vi "read_config_file.vi"(8 "error in (no error)":errorcluster, 10 "force load?":bool, 11 "StageMG100204SutterMP285 in":refnum<class "StageMG100204SutterMP285.lvclass">=refnum) -> (0 "error out":errorcluster, 3 "StageMG100204SutterMP285 out":refnum<class "StageMG100204SutterMP285.lvclass">)   [LabVIEW 2010, in "StageMG100204SutterMP285.lvclass"]
doc: "The dynamic dispatch version of this VI loads the config file from the config_files folder of the actual plug-in class. The name of the config file to be loaded is property of the plug-in object. If not explicitely set, a file config_files/config.xml is loaded by default."
uses:
  StageMG100204SutterMP285.lvclass
  configuration_data_cluster.ctl
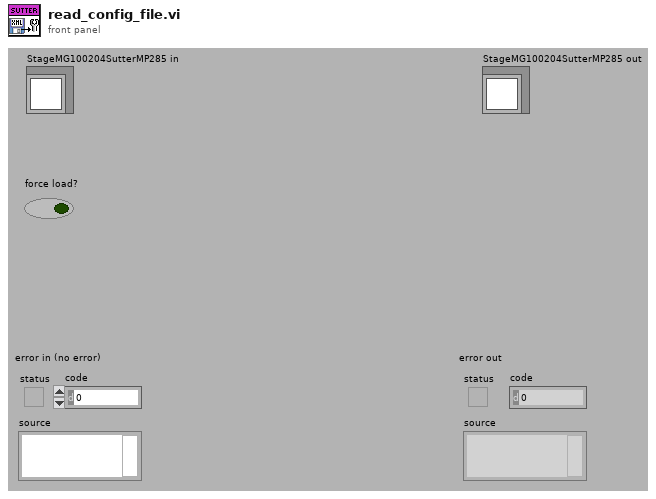
[diagram p1: front panel]
types:
  T1 = typedef "StageMG100204SutterMP285.lvclass/configuration_data_cluster.ctl" = cluster{"serial port":dbl, "HiRes Speed":dbl, "LoRes Speed":dbl}
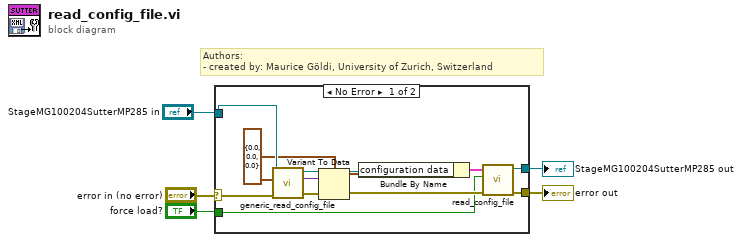
[diagram p0: block diagram]
diagram:
  # "Authors: \n- created by: Maurice Göldi, University of Zurich, Switzerland"
  n1 = case shown="No Error" "error in (no error)" {
    selector: "error in (no error)" -> [w10 w18]
    tunnel: [w15 w18] -> w4
    tunnel: [w14 w19] -> w1
    tunnel: "StageMG100204SutterMP285 in" -> [w7 w19]
    tunnel: "force load?" -> [w12 _]
    frame No Error {
      w6 = T1 {"serial port"=0.0, "HiRes Speed"=0.0, "LoRes Speed"=0.0} ("configuration data")
      n2 = call-dynamic "generic_read_config_file.vi"("error in (no error)"=w10, "config cluster variant in (data type)"=w6, "GenericPlugin in"=w7) -> ("error out"=w11:errorcluster, "config cluster variant out (populated"=w9:variant, "GenericPlugin out"=w8:refnum<class "StageMG100204SutterMP285.lvclass">)  [unwired: 6 in]
      n3 = Variant To Data(error in=w11, Variant=w9, type=w6) -> (error out=w16:errorcluster, data=w17:T1)
      n4 = Bundle By Name(cluster=w8, "configuration data"=w17) -> (w13:cluster{})
      n5 = call-parent "read_config_file.vi"("error in (no error)"=w16, "force load?"=w12, "GenericPlugin in"=w13) -> ("error out"=w15:errorcluster, "GenericPlugin out"=w14:refnum<class "StageMG100204SutterMP285.lvclass">)  [unwired: 7 in]
    }
    frame Error {
    }
  }
  "error out" <- w4
  "StageMG100204SutterMP285 out" <- w1
